vi "GetRoi.vi"() -> (1 "FirstCol":i32=512, 2 "RowBin":i32, 3 "LastCol":i32, 4 "FirstRow":i32, 5 "LastRow":i32, 6 "ColBin":i32=512)   [LabVIEW 2014]
panel:
  out "Error":bool
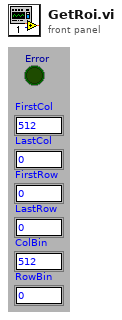
[diagram p1: front panel]
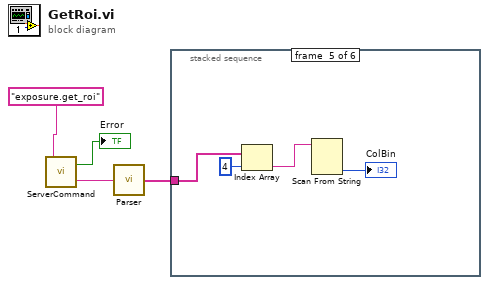
[diagram p0: block diagram]
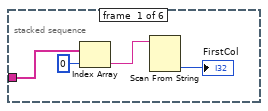
[diagram p2: hidden frame]
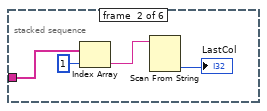
[diagram p3: hidden frame]
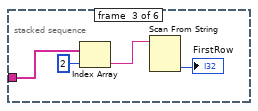
[diagram p4: hidden frame]
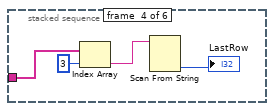
[diagram p5: hidden frame]
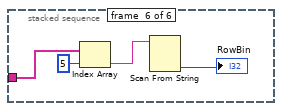
[diagram p6: hidden frame]
diagram:
  n1 = call "ServerCommand.vi"("Command"="exposure.get_roi") -> ("Error"=→"Error":bool, "Reply"=w3:string)
  n2 = call "Parser.vi"("string"=w3) -> ("Out Strings"=w1:string[])
  n3 = stacked-sequence {
    tunnel: w1 -> [w7 w12 w16 w20 w24 w28]
    frame #0 {
      n4 = Index Array(array=w7, index=0) -> (element=w5:string)
      n5 = Scan From String(input string=w5) -> (output 1=→"FirstCol":i32)  [unwired: 4 in, 3 out]
    }
    frame #1 {
      n6 = Index Array(array=w12, index=1) -> (element=w10:string)
      n7 = Scan From String(input string=w10) -> (output 1=→"LastCol":i32)  [unwired: 4 in, 3 out]
    }
    frame #2 {
      n8 = Index Array(array=w16, index=2) -> (element=w14:string)
      n9 = Scan From String(input string=w14) -> (output 1=→"FirstRow":i32)  [unwired: 4 in, 3 out]
    }
    frame #3 {
      n10 = Index Array(array=w20, index=3) -> (element=w18:string)
      n11 = Scan From String(input string=w18) -> (output 1=→"LastRow":i32)  [unwired: 4 in, 3 out]
    }
    frame #4 {
      n12 = Index Array(array=w24, index=4) -> (element=w22:string)
      n13 = Scan From String(input string=w22) -> (output 1=→"ColBin":i32)  [unwired: 4 in, 3 out]
    }
    frame #5 {
      n14 = Index Array(array=w28, index=5) -> (element=w26:string)
      n15 = Scan From String(input string=w26) -> (output 1=→"RowBin":i32)  [unwired: 4 in, 3 out]
    }
  }
